vi "Wheel(1).vi"() -> ()   [LabVIEW 2020]
uses:
  <vilib>/DAQmx/read.llb/DAQmx Read (Counter DBL 1Chan 1Samp).vi
  <vilib>/DAQmx/create/channels.llb/DAQmx Create Channel (CI-Position-Angular Encoder).vi
  Shared/Experiment/ExperimentGlobals.vi
  <vilib>/Utility/file.llb/Write Delimited Spreadsheet (string).vi
  Shared/ModuleCrosstalk/Crosstalk.vi
  <vilib>/DAQmx/miscellaneous.llb/DAQmx Fill In Error Info.vi
  <vilib>/Utility/file.llb/Write Delimited Spreadsheet (DBL).vi
panel:
  out "Numeric":i32
  out "Speed av. 1s(cm/s) 2":dbl
  out "Output file":path
  out "Speed (cm/s)":dbl
  out "Counter task":refnum<k21>
  out "Aquiering":bool
  out "Distance (m)":dbl
  out "Angle (deg)":dbl
  out "Motion plot":dbl(graph)
  out "Recording":bool
  # "Mouse Wheel"
  # "Wires (left-right) : black-empty-green-orange-yellow"
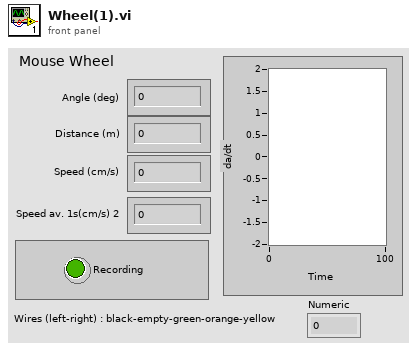
[diagram p1: front panel]
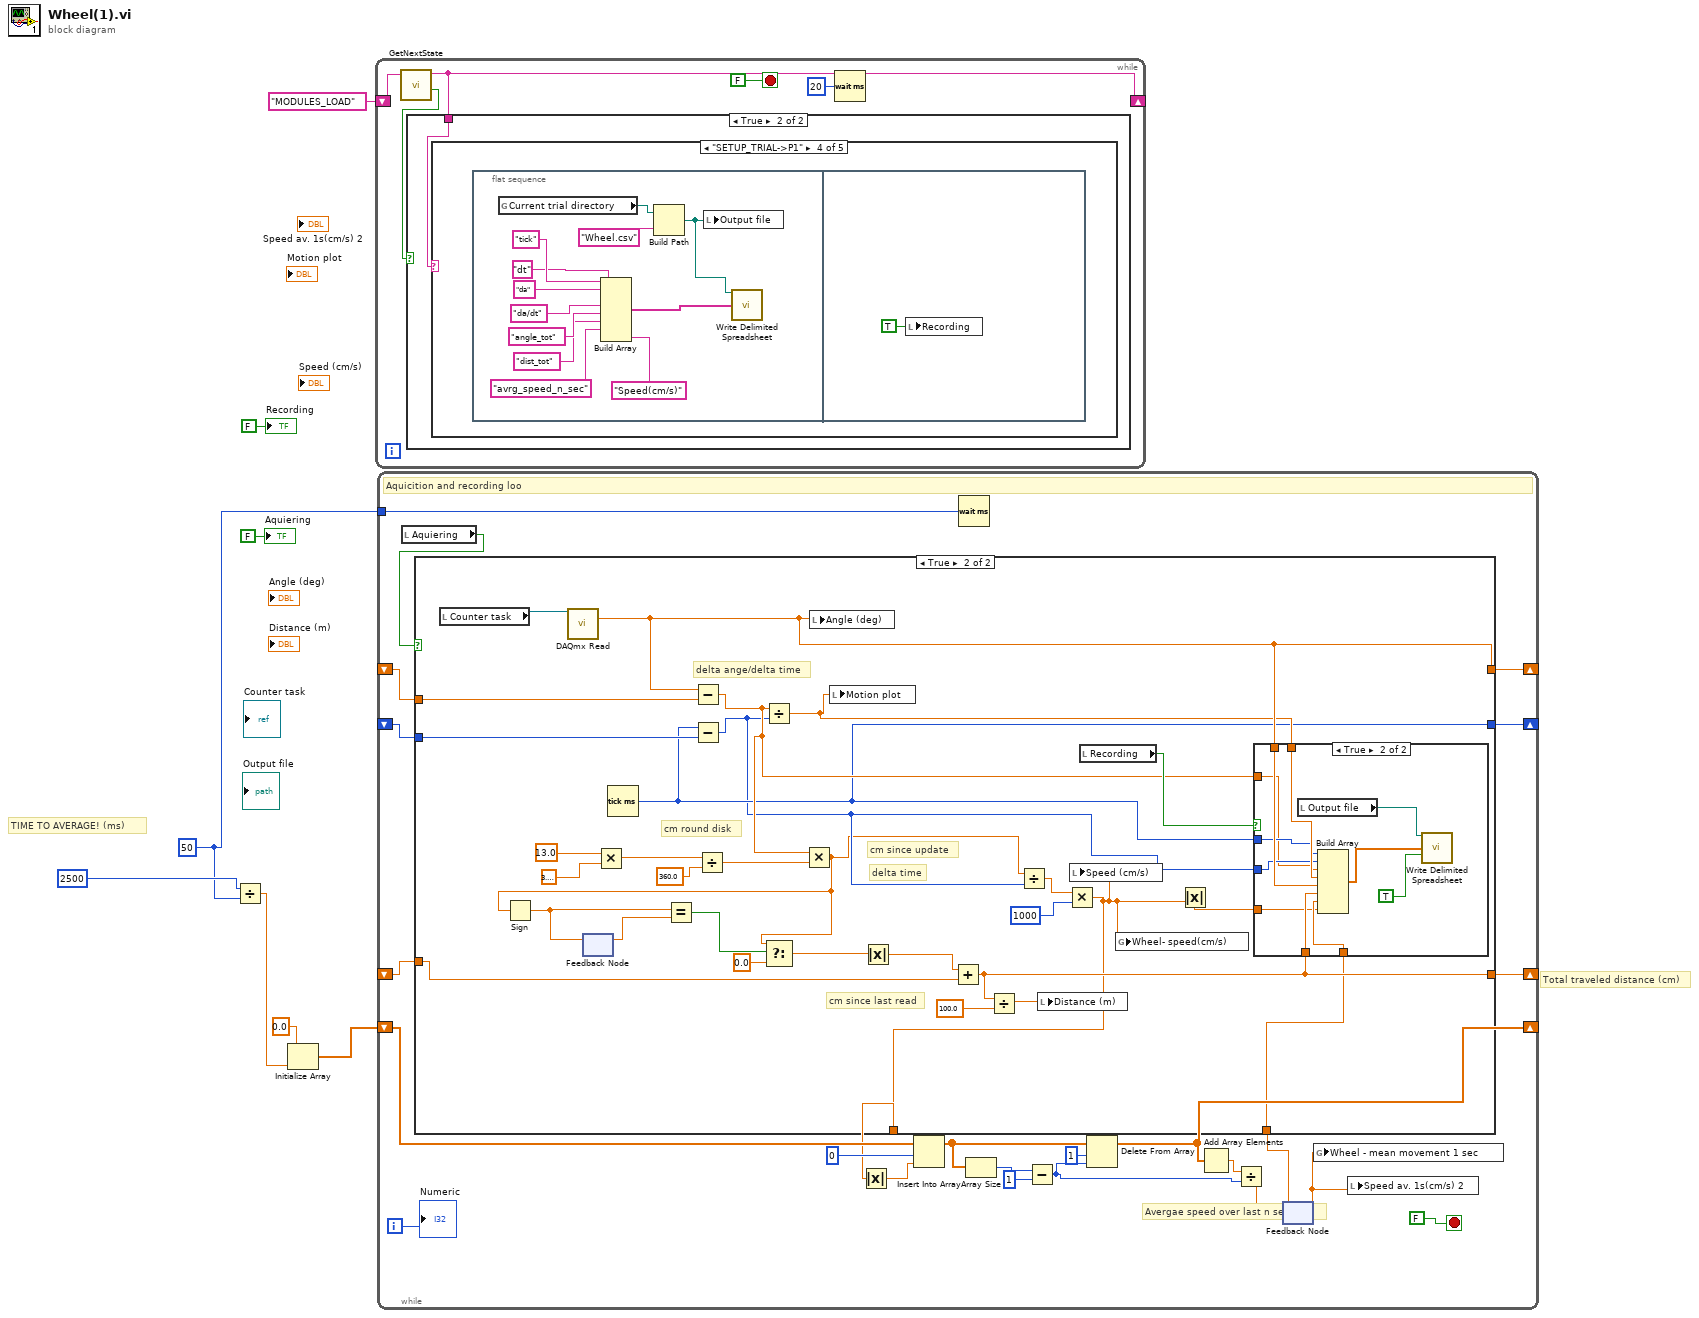
[diagram p0: block diagram]
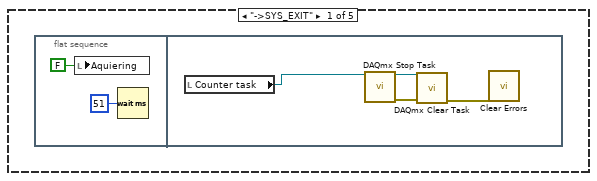
[diagram p5: hidden frame]
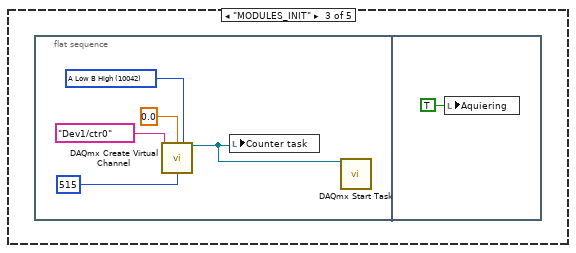
[diagram p7: hidden frame]
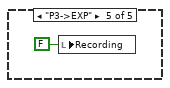
[diagram p8: hidden frame]
diagram:
  w4 = 50
  # "TIME TO AVERAGE! (ms)"
  # "Total traveled distance (cm)"
  n1 = Divide(x=2500, y=w4) -> (x/y=w3:dbl)
  n2 = Initialize Array(0.0, w3) -> (w1:dbl[])
  n3 = while {
    shift-right: [w9] -> _
    shift-left: "MODULES_LOAD" ("Next state") -> [w11]
    stop <- FALSE stop-if-true
    n4 = call "GetNextState.vi"("Current state"=w11) -> ("State has changed?"=w10:bool, "Next state"=w9:string)  [unwired: 9 in]
    n5 = case shown="True" w10 {
      tunnel: w9 -> [_ w14]
      frame False {
      }
      frame True {
        n6 = case shown="\"SETUP_TRIAL->P1\"" w14 {
          frame "->SYS_EXIT" {
            n7 = flat-sequence {
              frame #0 {
                n8 = local write "Aquiering"(FALSE ("Aquiering")) -> ()
                n9 = Wait (ms)(milliseconds to wait=u32 51) -> ()  [unwired: 1 out]
              }
              frame #1 {
                n10 = local read "Counter task"() -> (w17:refnum<k21>)
                n11 = call <vilib>:"DAQmx Stop Task.vi"("task/channels in"=w17) -> ("task out"=w18:refnum<k21>, "error out"=w19:errorcluster)  [unwired: 13 in]
                n12 = call <vilib>:"DAQmx Clear Task.vi"("task in"=w18, "error in"=w19) -> ("error out"=w20:errorcluster)  [unwired: 13 in]
                n13 = call <vilib>:"Clear Errors.vi"("error in (no error)"=w20) -> ()  [unwired: 5 in, 2 out]
              }
            }
          }
          frame Default {
          }
          frame "MODULES_INIT" {
            n14 = flat-sequence {
              frame #0 {
                w21 = 10042 items=["A High B High"=10040, "A High B Low"=10041, "A Low B High"=10042, "A Low B Low"=10043] ("z index phase")
                n15 = call-poly <vilib>:"DAQmx Create Virtual Channel.vi"("z index value"=0.0, "z index phase"=w21, "counter"=tag "Dev1/ctr0", "pulses per revolution"=u32 515) -> ("task out"=w23:refnum<k21>)  [unwired: 10 in, 1 out]
                n16 = local write "Counter task"(w23) -> ()
                n17 = call <vilib>:"DAQmx Start Task.vi"("task/channels in"=w23) -> ()  [unwired: 13 in, 2 out]
              }
              frame #1 {
                n18 = local write "Aquiering"(TRUE ("Aquiering")) -> ()
              }
            }
          }
          frame "SETUP_TRIAL->P1" {
            n19 = flat-sequence {
              frame #0 {
                n20 = global read "ExperimentGlobals.vi" "Current trial directory"() -> (w38:path)
                n21 = Build Array("tick", "dt" ("element"), "da" ("element"), "da/dt" ("element"), "angle_tot" ("element"), "dist_tot" ("element"), "avrg_speed_n_sec" ("element"), "Speed(cm/s)" ("element")) -> (w35:string[])
                n22 = Build Path(base path=w38, name or relative path="Wheel.csv") -> (appended path=w36:path)
                n23 = local write "Output file"(w36) -> ()
                n24 = call-poly <vilib>:"Write Delimited Spreadsheet.vi"("file path (dialog if empty)"=w36, "1D data"=w35) -> ()  [unwired: 12 in, 2 out]
              }
              frame #1 {
                n25 = local write "Recording"(TRUE ("Recording")) -> ()
              }
            }
          }
          frame "P3->EXP" {
            n26 = local write "Recording"(FALSE ("Recording")) -> ()
          }
        }
      }
    }
    n27 = Wait (ms)(milliseconds to wait=u32 20) -> ()  [unwired: 1 out]
  }
  n28 = while {
    shift-right: [w61] -> _
    shift-left: _ -> [w59]
    shift-right: [w60] -> _
    shift-left: _ -> [w58]
    shift-right: [w56] -> _
    shift-left: _ -> [w57]
    tunnel: w4 -> [w55]
    shift-right: [w47] -> _
    shift-left: w1 -> [w49]
    i -> [w48]
    stop <- FALSE stop-if-true
    # "Avergae speed over last n seconds"
    # "Aquicition and recording loo"
    n29 = local read "Aquiering"() -> (w63:bool)
    n30 = Wait (ms)(milliseconds to wait=w55) -> ()  [unwired: 1 out]
    n31 = feedback #1() -> (w41:dbl)  [unwired: 1 in]
    n32 = case shown="True" w63 {
      tunnel: [_ w82] -> w61
      tunnel: [_ w78] -> w60
      tunnel: w59 -> [_ w92]
      tunnel: w58 -> [_ w91]
      tunnel: w57 -> [_ w88]
      tunnel: [_ w80] -> w56
      tunnel: [_ w75] -> w43
      tunnel: w41 -> [_ w76]
      frame False {
      }
      frame True {
        # "delta time"
        # "cm since update"
        # "delta ange/delta time"
        # "cm since last read"
        # "cm round disk"
        n33 = local read "Counter task"() -> (w93:refnum<k21>)
        n34 = call-poly <vilib>:"DAQmx Read.vi"("task/channels in"=w93) -> ("data"=w82:dbl)  [unwired: 12 in, 2 out]
        n35 = feedback #2() -> (w64:dbl)  [unwired: 1 in]
        n36 = Multiply(x=13.0, y=3.141592653589793) -> (x*y=w71:dbl)
        n37 = Tick Count (ms)() -> (millisecond timer value=w78:u32)
        n38 = Subtract(x=w82, y=w92) -> (x-y=w79:dbl)
        n39 = Subtract(x=w78, y=w91) -> (x-y=w77:u32)
        n40 = Divide(x=w71, y=360.0) -> (x/y=w89:dbl)
        n41 = Divide(x=w79, y=w77) -> (x/y=w81:dbl)
        n42 = Multiply(x=w79, y=w89) -> (x*y=w66:dbl)
        n43 = Sign(1:w66) -> (0:w65:dbl)
        n44 = feedback-in #2(w65) -> ()
        n45 = Equal?(x=w65, y=w64) -> (x = y?=w70:bool)
        n46 = Select(t=w66, s=w70, f=0.0) -> (s? t:f=w68:dbl)
        n47 = local write "Angle (deg)"(w82) -> ()
        n48 = local write "Motion plot"(w81) -> ()
        n49 = Absolute Value(x=w68) -> (abs(x)=w67:dbl)
        n50 = Add(x=w67, y=w88) -> (x+y=w80:dbl)
        n51 = Divide(x=w80, y=100.0) -> (x/y=w87:dbl)
        n52 = Divide(x=w66, y=w77) -> (x/y=w84:dbl)
        n53 = local write "Distance (m)"(w87) -> ()
        n54 = Multiply(x=w84, y=u32 1000) -> (x*y=w75:dbl)
        n55 = local write "Speed (cm/s)"(w75) -> ()
        n56 = local read "Recording"() -> (w83:bool)
        n57 = global write "Crosstalk.vi" "Wheel- speed(cm/s)"(w75) -> ()
        n58 = Absolute Value(x=w75) -> (abs(x)=w74:dbl)
        n59 = case shown="True" w83 {
          tunnel: w78 -> [_ w98]
          tunnel: w82 -> [_ w100]
          tunnel: w81 -> [_ w101]
          tunnel: w77 -> [_ w97]
          tunnel: w80 -> [_ w99]
          tunnel: w79 -> [_ w96]
          tunnel: w76 -> [_ w95]
          tunnel: w74 -> [_ w94]
          frame False {
          }
          frame True {
            n60 = local read "Output file"() -> (w104:path)
            n61 = Build Array(w98, w97, w96, w101, w100, w99, w95, w94) -> (w102:dbl[])
            n62 = call-poly <vilib>:"Write Delimited Spreadsheet.vi"("file path (dialog if empty)"=w104, "1D data"=w102, "append to file? (new file:F)"=TRUE ("append to file? (F)")) -> ()  [unwired: 11 in, 2 out]
          }
        }
      }
    }
    n63 = Absolute Value(x=w43) -> (abs(x)=w44:dbl)
    n64 = Insert Into Array(array=w49, index=0, new element=w44) -> (w51:dbl[])
    n65 = Array Size(array=w51) -> (size(s)=w52:i32)
    n66 = Subtract(x=w52, y=1) -> (x-y=w45:i32)
    n67 = Delete From Array(array=w51, length=1, index=w45) -> (array with subset deleted=w47:dbl[])  [unwired: 1 out]
    n68 = Add Array Elements(numeric array=w47) -> (sum=w46:dbl)
    n69 = Divide(x=w46, y=w45) -> (x/y=w42:dbl)
    n70 = feedback-in #1(w42) -> ()
    n71 = global write "Crosstalk.vi" "Wheel - mean movement 1 sec"(w41) -> ()
    n72 = local write "Speed av. 1s(cm/s) 2"(w41) -> ()
    "Numeric" <- w48
  }
  "Recording" <- FALSE ("Recording")
  "Aquiering" <- FALSE ("Aquiering")
